vi "Python_Mainloop.vi"(8 "error in (no error)":errorcluster) -> (0 "error out":errorcluster)   [LabVIEW 2021]
doc: "This example demonstrates how to call a Python function and pass integers as arguments. It uses a python function to compute the sum of two integers."
uses:
  Global_Variables.vi
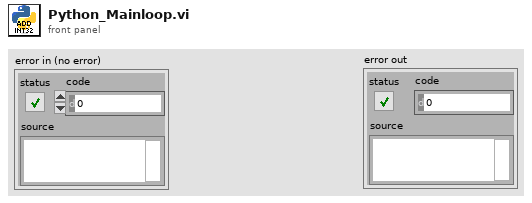
[diagram p1: front panel]
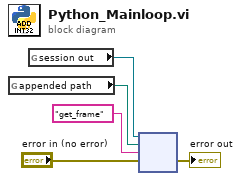
[diagram p0: block diagram]
diagram:
  n1 = global read "Global_Variables.vi" "appended path"() -> (w2:path)
  n2 = global read "Global_Variables.vi" "session out"() -> (w1:refnum<k35>)
  n3 = node(w1, w2, "get_frame" ("function name"), "error in (no error)") -> (→"error out":errorcluster)  [unwired: 2 in, 3 out]
